vi "Feedback_Sum.vi"() -> ()   [LabVIEW 2024]
panel:
  out "x+y":i32
  in  "Numeric":i32
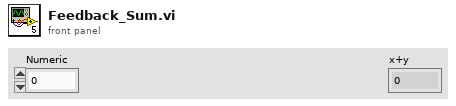
[diagram p1: front panel]
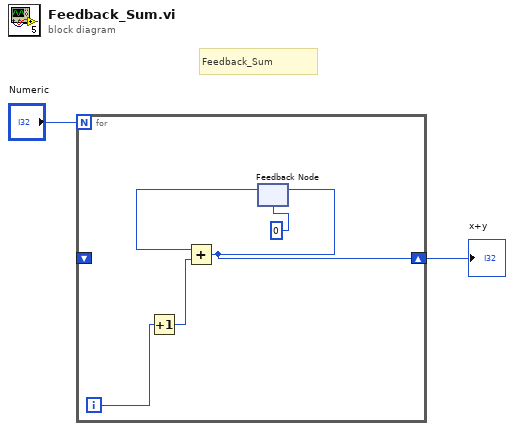
[diagram p0: block diagram]
diagram:
  # "Feedback_Sum"
  n1 = for {
    N: "Numeric" -> [_]
    shift-right: [w3] -> w1
    shift-left: _ -> [_]
    i -> [w7]
    n2 = Increment(x=w7) -> (x+1=w6:i32)
    n3 = feedback #1(0) -> (w5:i32)
    n4 = Add(x=w5, y=w6) -> (x+y=w3:i32)
    n5 = feedback-in #1(w3) -> ()
  }
  "x+y" <- w1
